vi "Update_Bearing_Temp_Clust.vi"(8 "error in (no error)":errorcluster, 10 "Data In":variant, 11 "MHL_Data In":T1) -> (0 "error out":errorcluster, 3 "MHL_Data out":T1)   [LabVIEW 2019, in "MHL.lvlib"]
uses:
  MHL.lvlib
  typedef/MHL_Data.ctl
  Alarm_Panel/Channel_Temperature_Threshold.ctl
  typedef/Alarm_Panel.ctl
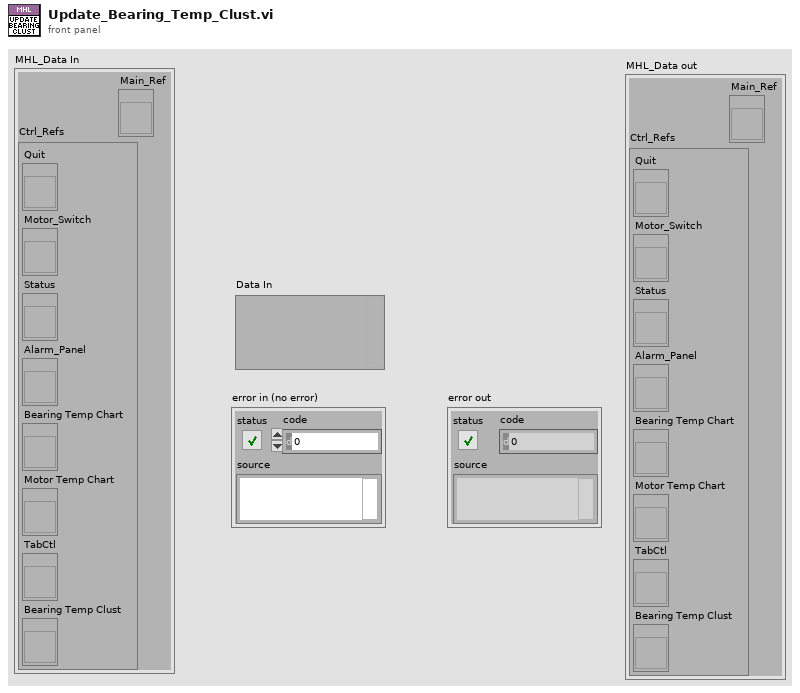
[diagram p1: front panel]
types:
  T1 = typedef "MHL.lvlib/MHL_Data.ctl" = cluster{"Ctrl_Refs":cluster{"Quit":refnum<vi>, "Motor_Switch":refnum<vi>, "Status":refnum<vi>, "Alarm_Panel":refnum<vi>, "Bearing Temp Chart":refnum<vi>, "Motor Temp Chart":refnum<vi>, "TabCtl":refnum<vi>, "Bearing Temp Clust":refnum<vi>}, "Main_Ref":refnum<vi>}
  T2 = typedef "Alarm_Panel.ctl" = cluster{"Channel (0 - 7)":cluster{"Channel Temperature Thresholds":T3, "Channel Temperature Thresholds 2":T3, "Channel Temperature Thresholds 3":T3, "Channel Temperature Thresholds 4":T3, "Channel Temperature Thresholds 5":T3, "Channel Temperature Thresholds 6":T3, "Channel Temperature Thresholds 7":T3, "Channel Temperature Thresholds 8":T3}, "Channel (8 - 15)":cluster{"Channel Temperature Thresholds":T3, "Channel Temperature Thresholds 2":T3, "Channel Temperature Thresholds 3":T3, "Channel Temperature Thresholds 4":T3, "Channel Temperature Thresholds 5":T3, "Channel Temperature Thresholds 6":T3, "Channel Temperature Thresholds 7":T3, "Channel Temperature Thresholds 8":T3}, "Channel (16 - 23)":cluster{"Channel Temperature Thresholds":T3, "Channel Temperature Thresholds 2":T3, "Channel Temperature Thresholds 3":T3, "Channel Temperature Thresholds 4":T3, "Channel Temperature Thresholds 5":T3, "Channel Temperature Thresholds 6":T3, "Channel Temperature Thresholds 7":T3, "Channel Temperature Thresholds 8":T3}, "Channel (24 - 31)":cluster{"Channel Temperature Thresholds":T3, "Channel Temperature Thresholds 2":T3, "Channel Temperature Thresholds 3":T3, "Channel Temperature Thresholds 4":T3, "Channel Temperature Thresholds 5":T3, "Channel Temperature Thresholds 6":T3, "Channel Temperature Thresholds 7":T3, "Channel Temperature Thresholds 8":T3}}
  T3 = typedef "Channel_Temperature_Threshold.ctl" = cluster{"Min":i32, "Max":i32, "Alarm":i32, "Status":u32}
  T4 = cluster{"Channel Temperature Thresholds":T3, "Channel Temperature Thresholds 2":T3, "Channel Temperature Thresholds 3":T3, "Channel Temperature Thresholds 4":T3, "Channel Temperature Thresholds 5":T3, "Channel Temperature Thresholds 6":T3, "Channel Temperature Thresholds 7":T3, "Channel Temperature Thresholds 8":T3}
  T5 = cluster{"Channel Temperature Thresholds":T3, "Channel Temperature Thresholds 2":T3, "Channel Temperature Thresholds 3":T3, "Channel Temperature Thresholds 4":T3, "Channel Temperature Thresholds 5":T3, "Channel Temperature Thresholds 6":T3, "Channel Temperature Thresholds 7":T3, "Channel Temperature Thresholds 8":T3}[]
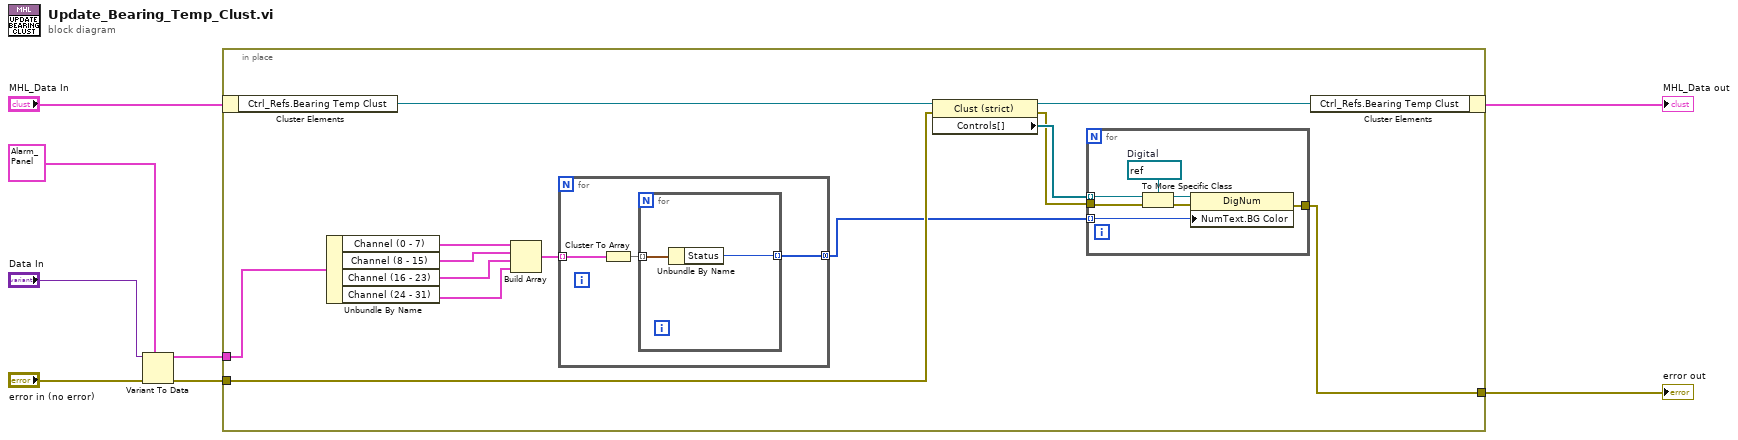
[diagram p0: block diagram]
diagram:
  n1 = Variant To Data(error in="error in (no error)", type=T2 {"Channel (0 - 7)"={"Channel Temperature Thresholds"={"Min"=0, "Max"=0, "Alarm"=0, "Status"=0}, "Channel Temperature Thresholds 2"={"Min"=0, "Max"=0, "Alarm"=0, "Status"=0}, "Channel Temperature Thresholds 3"={"Min"=0, "Max"=0, "Alarm"=0, "Status"=0}, "Channel Temperature Thresholds 4"={"Min"=0, "Max"=0, "Alarm"=0, "Status"=0}, "Channel Temperature Thresholds 5"={"Min"=0, "Max"=0, "Alarm"=0, "Status"=0}, "Channel Temperature Thresholds 6"={"Min"=0, "Max"=0, "Alarm"=0, "Status"=0}, "Channel Temperature Thresholds 7"={"Min"=0, "Max"=0, "Alarm"=0, "Status"=0}, "Channel Temperature Thresholds 8"={"Min"=0, "Max"=0, "Alarm"=0, "Status"=0}}, "Channel (8 - 15)"={"Channel Temperature Thresholds"={"Min"=0, "Max"=0, "Alarm"=0, "Status"=0}, "Channel Temperature Thresholds 2"={"Min"=0, "Max"=0, "Alarm"=0, "Status"=0}, "Channel Temperature Thresholds 3"={"Min"=0, "Max"=0, "Alarm"=0, "Status"=0}, "Channel Temperature Thresholds 4"={"Min"=0, "Max"=0, "Alarm"=0, "Status"=0}, "Channel Temperature Thresholds 5"={"Min"=0, "Max"=0, "Alarm"=0, "Status"=0}, "Channel Temperature Thresholds 6"={"Min"=0, "Max"=0, "Alarm"=0, "Status"=0}, "Channel Temperature Thresholds 7"={"Min"=0, "Max"=0, "Alarm"=0, "Status"=0}, "Channel Temperature Thresholds 8"={"Min"=0, "Max"=0, "Alarm"=0, "Status"=0}}, "Channel (16 - 23)"={"Channel Temperature Thresholds"={"Min"=0, "Max"=0, "Alarm"=0, "Status"=0}, "Channel Temperature Thresholds 2"={"Min"=0, "Max"=0, "Alarm"=0, "Status"=0}, "Channel Temperature Thresholds 3"={"Min"=0, "Max"=0, "Alarm"=0, "Status"=0}, "Channel Temperature Thresholds 4"={"Min"=0, "Max"=0, "Alarm"=0, "Status"=0}, "Channel Temperature Thresholds 5"={"Min"=0, "Max"=0, "Alarm"=0, "Status"=0}, "Channel Temperature Thresholds 6"={"Min"=0, "Max"=0, "Alarm"=0, "Status"=0}, "Channel Temperature Thresholds 7"={"Min"=0, "Max"=0, "Alarm"=0, "Status"=0}, "Channel Temperature Thresholds 8"={"Min"=0, "Max"=0, "Alarm"=0, "Status"=0}}, "Channel (24 - 31)"={"Channel Temperature Thresholds"={"Min"=0, "Max"=0, "Alarm"=0, "Status"=0}, "Channel Temperature Thresholds 2"={"Min"=0, "Max"=0, "Alarm"=0, "Status"=0}, "Channel Temperature Thresholds 3"={"Min"=0, "Max"=0, "Alarm"=0, "Status"=0}, "Channel Temperature Thresholds 4"={"Min"=0, "Max"=0, "Alarm"=0, "Status"=0}, "Channel Temperature Thresholds 5"={"Min"=0, "Max"=0, "Alarm"=0, "Status"=0}, "Channel Temperature Thresholds 6"={"Min"=0, "Max"=0, "Alarm"=0, "Status"=0}, "Channel Temperature Thresholds 7"={"Min"=0, "Max"=0, "Alarm"=0, "Status"=0}, "Channel Temperature Thresholds 8"={"Min"=0, "Max"=0, "Alarm"=0, "Status"=0}}} ("Alarm Panel"), Variant="Data In") -> (data=w3:T2, error out=w4:errorcluster)
  n2 = in-place {
    in-place-border: w4 -> [w18]
    in-place-border: w3 -> [w17]
    in-place-border: [w9] -> w2
    n3 = in-place-cluster #1("MHL_Data In") -> ("Ctrl_Refs.Bearing Temp Clust"=w21:refnum<vi>)
    n4 = Unbundle By Name(w17) -> ("Channel (0 - 7)"=w16:T4, "Channel (8 - 15)"=w15:T4, "Channel (16 - 23)"=w14:T4, "Channel (24 - 31)"=w13:T4)
    n5 = Build Array(w16, w15, w14, w13) -> (w12:T5)
    n6 = for {
      tunnel: w12 -> [w24] mode=indexing
      tunnel: [w22] -> w11 mode=concatenating
      n7 = Cluster To Array(cluster=w24) -> (array=w23:T3[])
      n8 = for {
        tunnel: w23 -> [w26] mode=indexing
        tunnel: [w25] -> w22 mode=indexing
        n9 = Unbundle By Name(w26) -> ("Status"=w25:u32)
      }
    }
    n10 = property class="Clust (strict)"(reference=w21, error in=w18) -> (reference out=w10:refnum<vi>, error out=w19:errorcluster, "Controls[]"=w20:refnum<vi>[])
    n11 = for {
      tunnel: w20 -> [w33] mode=indexing
      tunnel: w19 -> [w31]
      tunnel: w11 -> [w28] mode=indexing
      tunnel: [w27] -> w9
      w32 = refnum<vi> refnum  # Digital
      n12 = To More Specific Class(target class=w32, reference=w33, error in=w31) -> (specific class reference=w30:refnum<vi>, error out=w29:errorcluster)
      n13 = property class="DigNum"(reference=w30, error in=w29, "NumText.BG Color"=w28) -> (error out=w27:errorcluster)  [unwired: 1 out]
    }
    n14 = in-place-cluster #1("Ctrl_Refs.Bearing Temp Clust"=w10) -> (→"MHL_Data out":T1)
  }
  "error out" <- w2
